vi "Barrier Attr Init.vi"(8 "error in (no error)":errorcluster, 11 "Barrier Attr in":T1) -> (0 "error out":errorcluster, 3 "Barrier Attr out":T1)   [LabVIEW 2016, in "Linux RT IPC.POSIX Threads.lvlib" / "Barrier Attr.lvclass"]
doc: "Calls pthread_barrierattr_init() on the pthread barrier attribute object encapsulated by Barrier Attr.\n\nThis VI initializes the barrier attribute object and sets its default values.\n\nRefer to online POSIX documentation for more information."
uses:
  Barrier Attr.lvclass
  Controls/reference.ctl
  C:/Git/SourceTree/LinuxRT-IPC/Source/POSIX Threads/Classes/POSIX Thread Object/POSIX Thread Object.lvclass
  POSIX Thread Object/POSIX Thread Object.lvclass/POSIX Thread Object.ctl
  POSIX Thread Object/Private VIs/libpthread path.vi
  POSIX Thread Object/Private VIs/get pthread error.vi
  POSIX Thread Object/POSIX Thread Object.lvclass
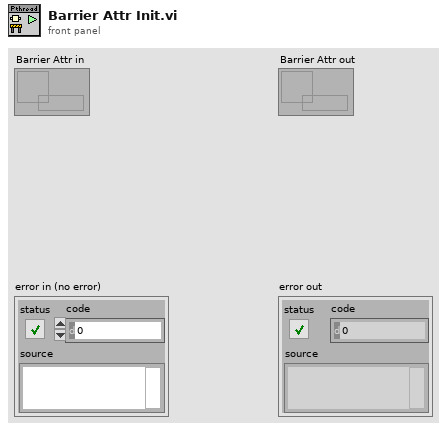
[diagram p1: front panel]
types:
  T1 = typedef "Linux RT IPC.POSIX Threads.lvlib/Barrier Attr.lvclass/reference.ctl" = refnum<data-value>
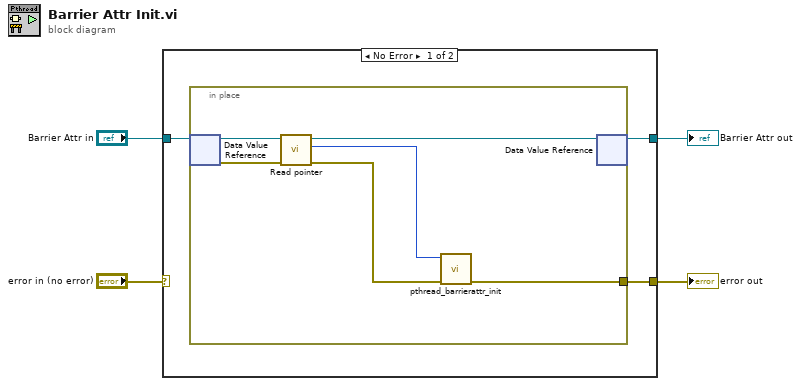
[diagram p0: block diagram]
diagram:
  n1 = case shown="No Error" "error in (no error)" {
    selector: "error in (no error)" -> [_ w15]
    tunnel: [w6 w15] -> w4
    tunnel: [w7 w14] -> w3
    tunnel: "Barrier Attr in" -> [w5 w14]
    frame No Error {
      n2 = in-place {
        in-place-border: [w11] -> w6
        n3 = in-place-dvr #1(w5) -> (w13:refnum<class "Barrier Attr.lvclass">, w9:errorcluster)
        n4 = call "Read pointer.vi"("error in (no error)"=w9, "POSIX Thread Object in"=w13) -> ("error out"=w8:errorcluster, "pointer"=w10:u64, "POSIX Thread Object out"=w12:refnum<class "Barrier Attr.lvclass">)  [unwired: 7 in]
        n5 = call "pthread_barrierattr_init.vi"("error in (no error)"=w8, "barrier attr ptr in"=w10) -> ("error out"=w11:errorcluster)  [unwired: 8 in, 1 out]
        n6 = in-place-dvr #1(w12) -> (w7:T1)  [unwired: 1 out]
      }
    }
    frame Error {
    }
  }
  "Barrier Attr out" <- w3
  "error out" <- w4
